vi "Stop.vi"(8 "error in (no error)":errorcluster, 11 "AdbBridge in":refnum<class "Adb Bridge.lvclass">) -> (0 "error out":errorcluster, 3 "AdbBridge out":refnum<class "Adb Bridge.lvclass">)   [LabVIEW 2016, in "Adb Bridge.lvclass"]
uses:
  Adb Bridge.lvclass
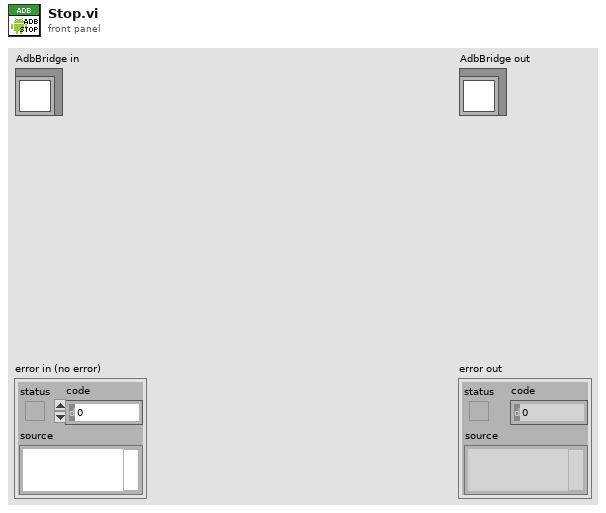
[diagram p1: front panel]
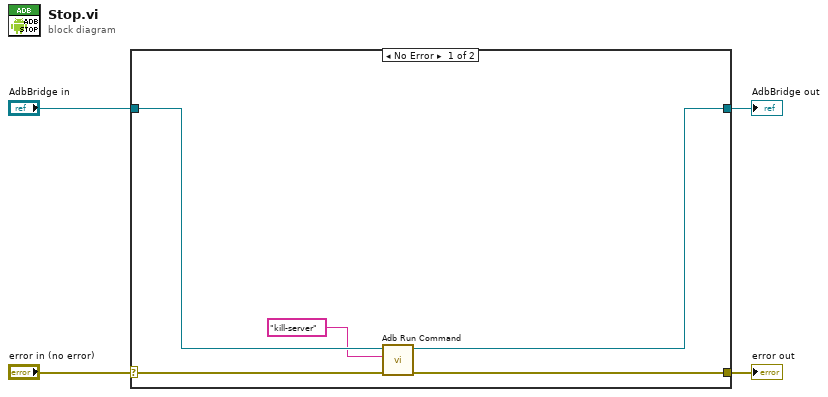
[diagram p0: block diagram]
diagram:
  n1 = case shown="No Error" "error in (no error)" {
    selector: "error in (no error)" -> [w6 w11]
    tunnel: [w5 w11] -> w3
    tunnel: [w8 w10] -> w1
    tunnel: "AdbBridge in" -> [w9 w10]
    frame No Error {
      n2 = call "Adb Run Command.vi"("error in (no error)"=w6, "args"="kill-server", "AdbBridge in"=w9) -> ("error out"=w5:errorcluster, "AdbBridge out"=w8:refnum<class "Adb Bridge.lvclass">)  [unwired: 7 in]
    }
    frame Error {
    }
  }
  "error out" <- w3
  "AdbBridge out" <- w1
